vi "Debouncing.vi"(10 "Cycles to Filter":u16=5, 11 "New Input Signal":bool) -> (2 "Signal Changed?":bool, 3 "New Signal":bool)   [LabVIEW 2021]
doc: "This VI compares the new input signal to the current output signal and looks for a change in state."
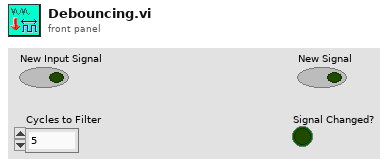
[diagram p1: front panel]
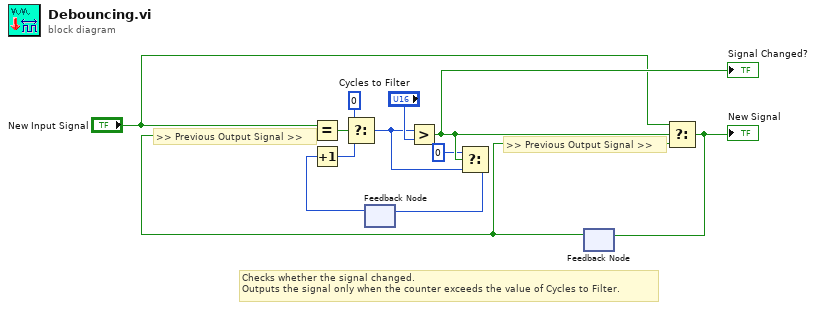
[diagram p0: block diagram]
diagram:
  # "Checks whether the signal changed.\nOutputs the signal only when the counter exceeds the value of Cycles to Filter."
  # ">> Previous Output Signal >>"
  # ">> Previous Output Signal >>"
  n1 = feedback #1() -> (w12:u16)  [unwired: 1 out]
  n2 = Increment(x=w12) -> (x+1=w7:u16)
  n3 = feedback #2() -> (w9:bool)  [unwired: 1 out]
  n4 = Equal?(x="New Input Signal", y=w9) -> (x = y?=w10:bool)
  n5 = Select(t=u16 0 ("f"), s=w10, f=w7) -> (s? t:f=w4:u16)
  n6 = Greater?(x=w4, y="Cycles to Filter") -> (0:w6:bool)
  "Signal Changed?" <- w6
  n7 = Select(t=u16 0, s=w6, f=w4) -> (s? t:f=w5:u16)
  n8 = feedback-in #1(w5) -> ()
  n9 = Select(t="New Input Signal", s=w6, f=w9) -> (s? t:f=w1:bool)
  "New Signal" <- w1
  n10 = feedback-in #2(w1) -> ()
